vi "Read Active Stop Conditions.vi"(1 "Active Stop Conditions":T1) -> (0 "Active Stop Conditions":T2[](array[typedef]))   [LabVIEW 2020, in "Iterator Actor.lvlib" / "Iterator Actor.lvclass"]
uses:
  Iterator Actor.lvclass
  Iterator Actor.lvclass/Iterator Actor.ctl
  Stop Condition.ctl
  Active Stop Conditions.ctl
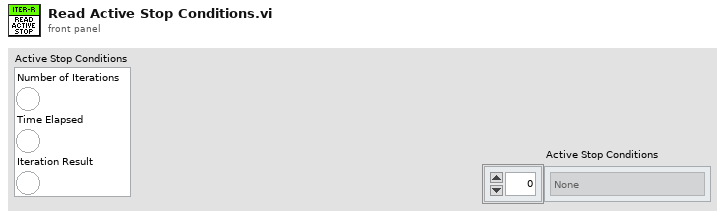
[diagram p1: front panel]
types:
  T1 = typedef "Iterator Actor.lvlib/Iterator Actor.lvclass/Active Stop Conditions.ctl" = cluster{"Number of Iterations":bool, "Time Elapsed":bool, "Iteration Result":bool}
  T2 = typedef "Iterator Actor.lvlib/Iterator Actor.lvclass/Stop Condition.ctl" = enum16{"None", "Number of Iterations", "Time Elapsed", "Iteration Result"}
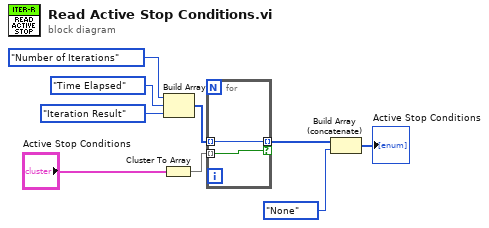
[diagram p0: block diagram]
diagram:
  n1 = Cluster To Array(cluster="Active Stop Conditions") -> (array=w8:bool[])
  n2 = Build Array(Stop_Condition."Number of Iterations" ("Stop Condition"), Stop_Condition."Time Elapsed" ("Stop Condition"), Stop_Condition."Iteration Result" ("Stop Condition")) -> (w4:T2[])
  n3 = for {
    tunnel: w8 -> [w10] mode=indexing
    tunnel: [w11] -> w3 mode=indexing if=w10
    tunnel: w4 -> [w11] mode=indexing
  }
  n4 = Build Array (concatenate)(w3, Stop_Condition."None" ("Stop Condition")) -> (→"Active Stop Conditions":T2[])
